vi "Configure PLL.vi"(7 "index":i32, 8 "error in":errorcluster, 10 "config":T1, 11 "fpga session in":refnum<k20>) -> (0 "error out":errorcluster, 3 "fpga session out":refnum<k20>)   [LabVIEW 2018, in "Lock-In Amplifier Example Host.lvlib"]
uses:
  Lock-In Amplifier Example Host.lvlib
  pll settings.ctl
  fpga type.ctl
  <vilib>/Utility/error.llb/Error Cluster From Error Code.vi
  <vilib>/rvi/errors/niLvFpgaAdjustHostInterfaceError.vi
  <vilib>/rvi/interface/nirviReadWriteControl/nirviReadWriteControl.xnode
  NiFpgaLv.dll
  <vilib>/rvi/interface/Simulation/niFpgaSimulationCallBeginRW.vi
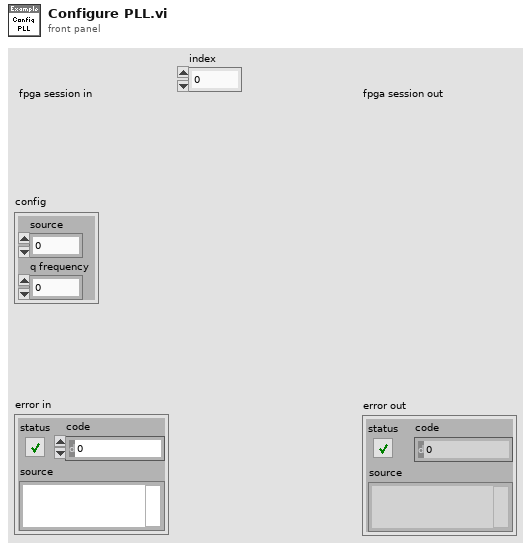
[diagram p1: front panel]
types:
  T1 = typedef "Lock-In Amplifier Example Host.lvlib/pll settings.ctl" = cluster{"source":i32, "q frequency":dbl}
  T2 = cluster{"quiescent frequency":fxp<+/-,48,0>, "compensation":fxp<+/-,18,3>, "psd gain":i16, "loop filter":cluster{"order":i32, "cutoff":i8}}
  T3 = typedef "Lock-In Amplifier Example Host.lvlib/fpga type.ctl" = refnum<k20>
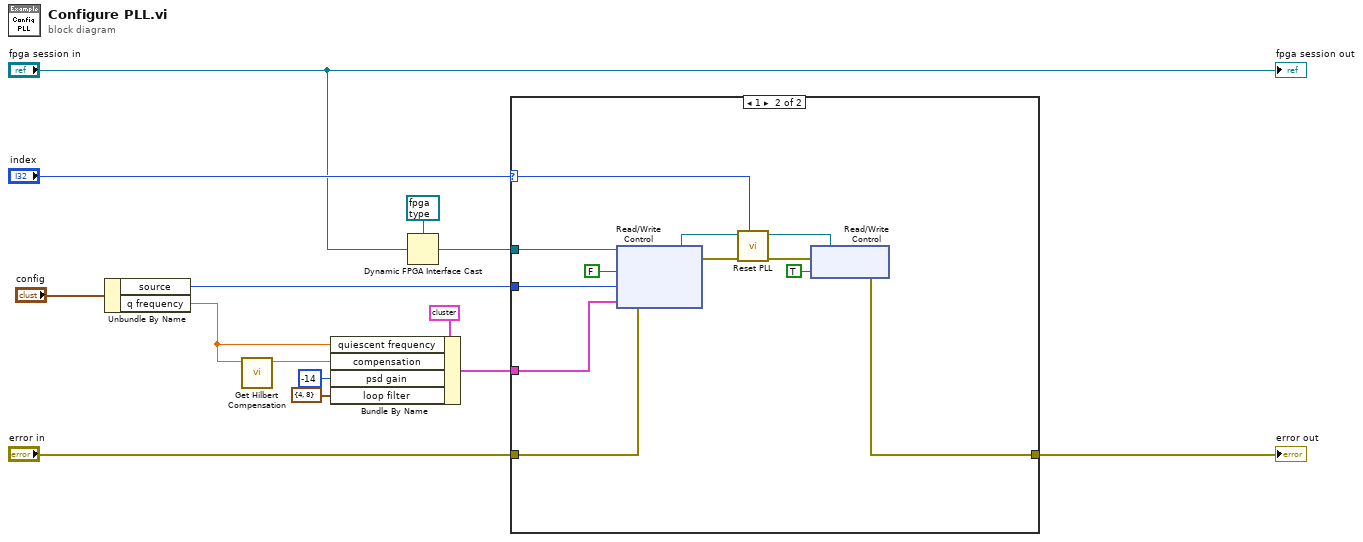
[diagram p0: block diagram]
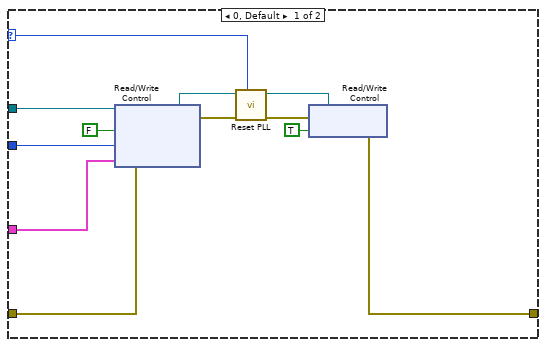
[diagram p2: hidden frame]
diagram:
  n1 = Unbundle By Name("config") -> ("source"=w2:i32, "q frequency"=w3:dbl)
  n2 = call "Get Hilbert Compensation.vi"("frequency"=w3) -> ("compensation value"=w4:dbl)  [unwired: 10 in]
  n3 = Bundle By Name(cluster=T2 {"quiescent frequency"=0.0, "compensation"=0.0, "psd gain"=0, "loop filter"={"order"=0, "cutoff"=0}} ("pll.config 0"), "quiescent frequency"=w3, "compensation"=w4, "psd gain"=i16 -14, "loop filter"=cluster{"order":i32, "cutoff":i8} {"order"=4, "cutoff"=8}) -> (w1:T2)
  n4 = Dynamic FPGA Interface Cast(Session In=T3 refnum ("fpga type"), Type="fpga session in") -> (Session Out=w12:T3)
  n5 = case shown="1" "index" {
    selector: "index" -> [w21 w33]
    tunnel: w12 -> [w26 w38]
    tunnel: [w16 w28] -> w11
    tunnel: "error in" -> [w24 w36]
    tunnel: w2 -> [w23 w35]
    tunnel: w1 -> [w22 w34]
    frame 0, Default {
      n6 = xnode "Read/Write Control"("FPGA VI Reference In"=w26, "error in"=w24, "pll.enable 0"=FALSE ("pll.enable 1"), "pll.channel 0"=w23, "pll.config 0"=w22) -> ("FPGA VI Reference Out"=w20:T3, "error out"=w19:errorcluster)
      n7 = call "Reset PLL.vi"("index"=w21, "error in"=w19, "fpga session in"=w20) -> ("error out"=w18:errorcluster, "fpga session out"=w17:T3)  [unwired: 7 in]
      n8 = xnode "Read/Write Control"("FPGA VI Reference In"=w17, "error in"=w18, "pll.enable 0"=TRUE ("pll.enable 1")) -> ("error out"=w16:errorcluster)  [unwired: 1 out]
    }
    frame 1 {
      n9 = xnode "Read/Write Control"("FPGA VI Reference In"=w38, "error in"=w36, "pll.enable 1"=FALSE, "pll.channel 1"=w35, "pll.config 1"=w34) -> ("FPGA VI Reference Out"=w32:T3, "error out"=w31:errorcluster)
      n10 = call "Reset PLL.vi"("index"=w33, "error in"=w31, "fpga session in"=w32) -> ("error out"=w30:errorcluster, "fpga session out"=w29:T3)  [unwired: 7 in]
      n11 = xnode "Read/Write Control"("FPGA VI Reference In"=w29, "error in"=w30, "pll.enable 1"=TRUE) -> ("error out"=w28:errorcluster)  [unwired: 1 out]
    }
  }
  "error out" <- w11
  "fpga session out" <- "fpga session in"
